vi "Send tt20panel_connect.vi"(7 "Message Priority (Normal)":T4=enum."Normal", 8 "error in (no error)":errorcluster, 9 "tt20_settings":T1, 10 "tt20_events":T3, 11 "Message Enqueuer":refnum<class "Message Enqueuer.lvclass">) -> (0 "error out":errorcluster, 3 "Message Enqueuer out":refnum<class "Message Enqueuer.lvclass">)   [LabVIEW 2015, in "tt20panel_connect Msg.lvclass"]
doc: "This VI sends the message to an actor."
uses:
  tt20panel_connect Msg.lvclass
  <vilib>/ActorFramework/Message Enqueuer/Message Enqueuer.lvclass
  <vilib>/ActorFramework/Message Enqueuer/Message Priority.ctl
  tt20panel_class/tt20_event_tdef.ctl
  tt20_class/tt20_hardware_info_tdef.ctl
  tt20panel_class/tt20_acq_mode_tdef.ctl
  tt20panel_connect Msg.lvclass/tt20panel_connect Msg.ctl
  <vilib>/ActorFramework/Message Enqueuer/Message Enqueuer.lvclass/Message Enqueuer.ctl
  <vilib>/ActorFramework/Message Priority Queue/Priority Enqueue.vi
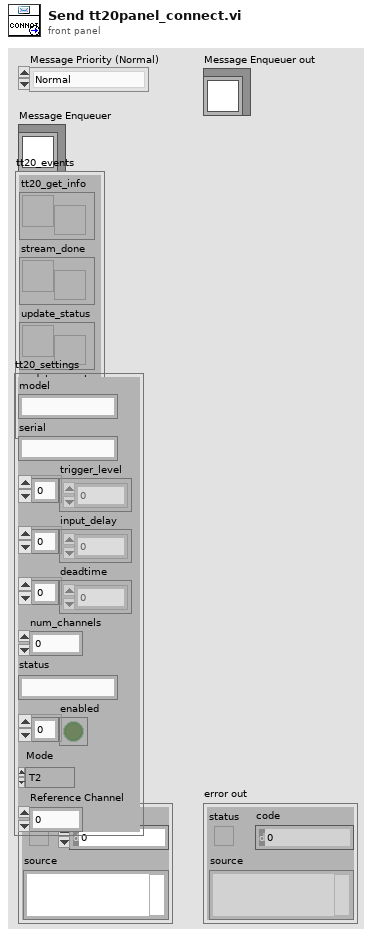
[diagram p1: front panel]
types:
  T1 = typedef "tt20_hardware_info_tdef.ctl" = cluster{"model":string, "serial":string, "trigger_level":dbl[], "input_delay":i64[], "deadtime":i64[], "num_channels":u32, "status":string, "enabled":bool[], "Mode":T2, "Reference Channel":u8}
  T2 = typedef "tt20_acq_mode_tdef.ctl" = enum16{"T2", "T3"}
  T3 = typedef "tt20_event_tdef.ctl" = cluster{"tt20_get_info":refnum<user-event>, "stream_done":refnum<user-event>, "update_status":refnum<user-event>, "update_counts":refnum<user-event>}
  T4 = typedef "Actor Framework.lvlib/Message Enqueuer.lvclass/Message Priority.ctl" = enum16{"Low", "Normal", "High"}
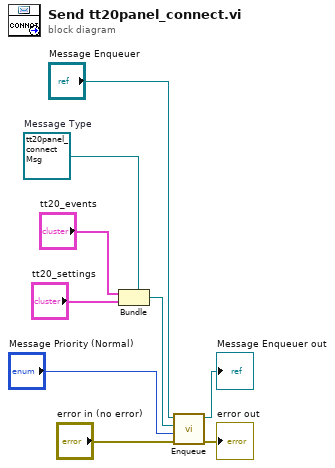
[diagram p0: block diagram]
diagram:
  w6 = refnum<class "tt20panel_connect Msg.lvclass"> refnum  # Message Type
  n1 = Bundle(cluster=w6, "tt20_events", "tt20_settings") -> (w5:refnum<class "tt20panel_connect Msg.lvclass">)
  n2 = call <vilib>:"Enqueue.vi"("error in (no error)"="error in (no error)", "Message Priority (Normal)"="Message Priority (Normal)", "Message"=w5, "Message Enqueuer in"="Message Enqueuer") -> ("error out"=→"error out":errorcluster, "Message Enqueuer out"=→"Message Enqueuer out":refnum<class "Message Enqueuer.lvclass">)  [unwired: 6 in]
